vi "Load Param ID Map.vi"(8 "error in (no error)":errorcluster, 11 "Param Id File in":path) -> (0 "error out":errorcluster, 2 "Param ID map":map{i32, string}(c390), 3 "Param Id File out":path)   [LabVIEW 2020, in "Ballard 1553 System Explorer.lvlib"]
uses:
  Ballard 1553 System Explorer.lvlib
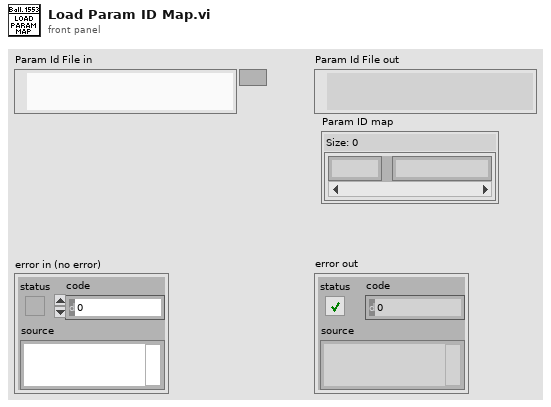
[diagram p1: front panel]
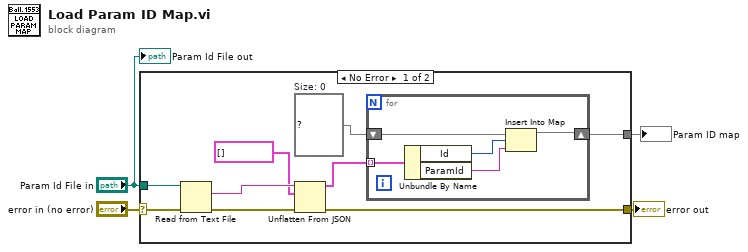
[diagram p0: block diagram]
diagram:
  n1 = case shown="No Error" "error in (no error)" {
    selector: "error in (no error)" -> [w12 w19]
    tunnel: "Param Id File in" -> [w13 _]
    tunnel: [w9 w19] -> w2
    tunnel: [w5 _] -> w1
    frame No Error {
      w6 = map{i32, string} {}  # Size: 0
      n2 = Read from Text File(file (use dialog)=w13, error in=w12) -> (text=w10:string, error out=w11:errorcluster)  [unwired: 2 in, 2 out]
      n3 = Unflatten From JSON(JSON string=w10, type and defaults=cluster{"Id":i32, "ParamId":string}[] [], error in (no error)=w11) -> (value=w7:cluster{"Id":i32, "ParamId":string}[], error out=w9:errorcluster)  [unwired: 4 in]
      n4 = for {
        tunnel: w7 -> [w18] mode=indexing
        shift-right: [w15] -> w5
        shift-left: w6 -> [w17]
        n5 = Unbundle By Name(w18) -> ("Id"=w16:i32, "ParamId"=w14:string)
        n6 = Insert Into Map(map in=w17, key=w16, value=w14) -> (map out=w15:map{i32, string})  [unwired: 2 out]
      }
    }
    frame Error {
    }
  }
  "error out" <- w2
  "Param ID map" <- w1
  "Param Id File out" <- "Param Id File in"
